vi "KeyboardSimulationForStringInput.vi"(0 "VI Reference In":refnum<vi>, 5 "Control Path":string, 7 "String Value":string, 11 "Error In":errorcluster) -> (4 "VI Reference Out":refnum<vi>, 15 "Error Out":errorcluster)   [LabVIEW 2016, in "Drona.lvlib" / "KeyboardSimulation.lvlib"]
doc: "Convert the input string value into key array and handle the actions configured for each of the keys in the control.\n\nThe input control name is given as a string , incase of path, use delimiters inbetween the path."
uses:
  KeyboardSimulation.lvlib
  typedef/VirtualKey.ctl
  typedef/Action.ctl
  user32.dll
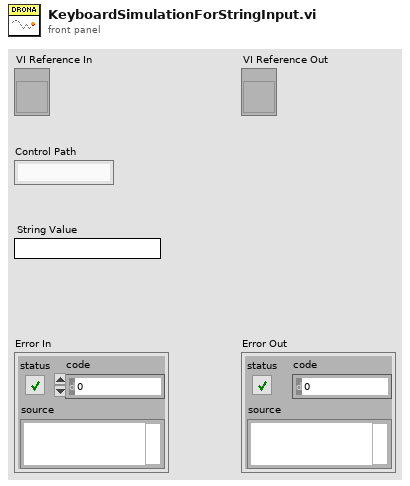
[diagram p1: front panel]
types:
  T1 = typedef "Drona.lvlib/KeyboardSimulation.lvlib/VirtualKey.ctl" = u8
  T2 = typedef "Drona.lvlib/KeyboardSimulation.lvlib/Action.ctl" = enum16{"Press", "Up", "Down"}
  T3 = cluster{"Key":T1, "Action":T2, "Delay (ms)":u32}[]
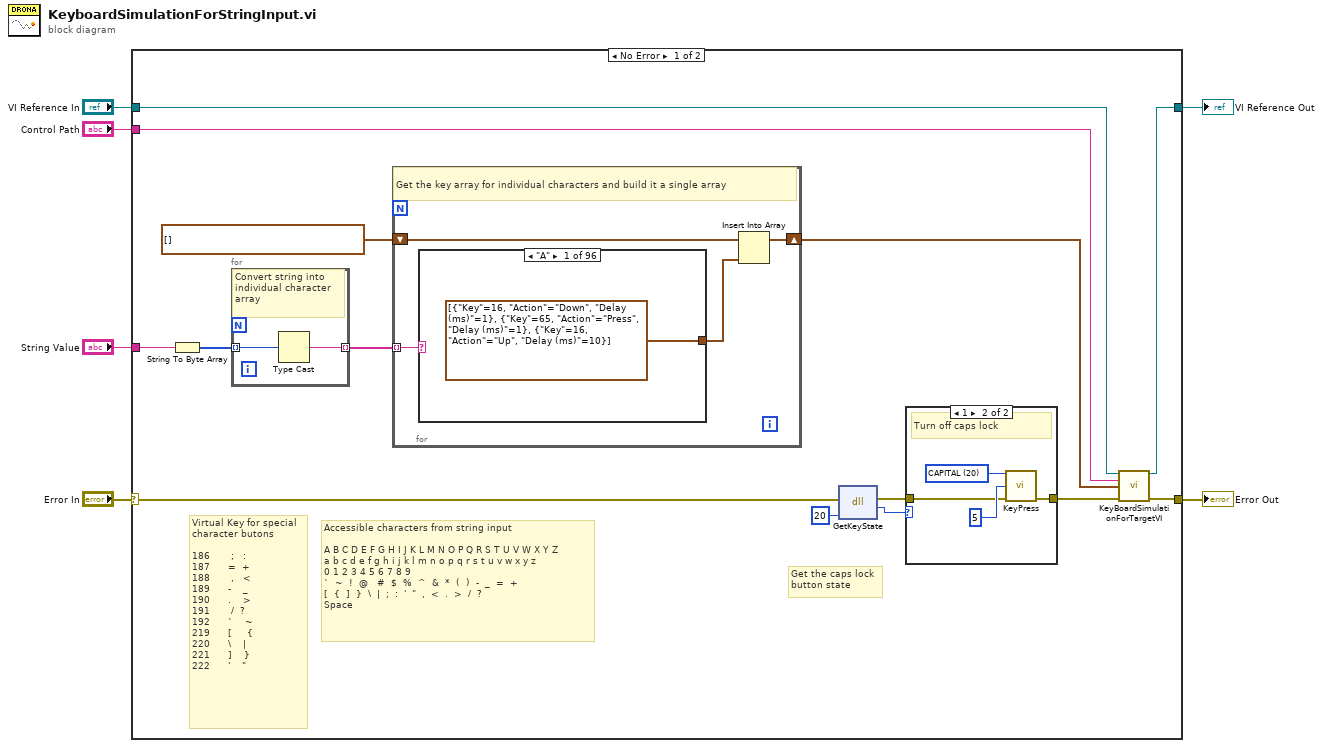
[diagram p0: block diagram]
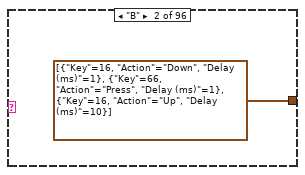
[diagram p2: hidden frame]
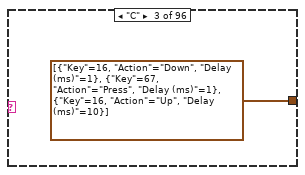
[diagram p3: hidden frame]
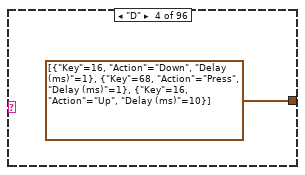
[diagram p4: hidden frame]
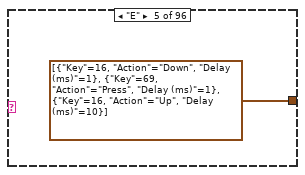
[diagram p5: hidden frame]
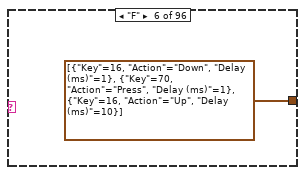
[diagram p6: hidden frame]
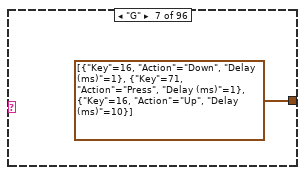
[diagram p7: hidden frame]
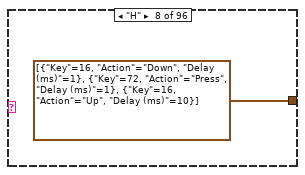
[diagram p8: hidden frame]
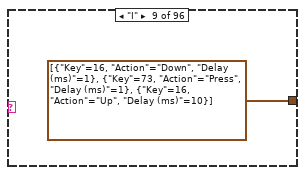
[diagram p9: hidden frame]
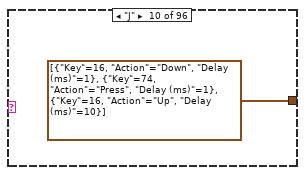
[diagram p10: hidden frame]
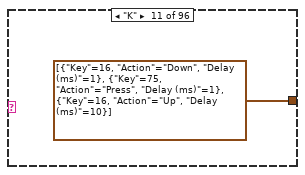
[diagram p11: hidden frame]
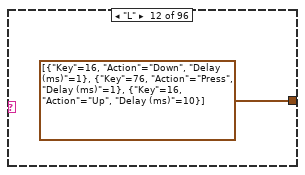
[diagram p12: hidden frame]
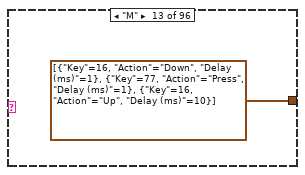
[diagram p13: hidden frame]
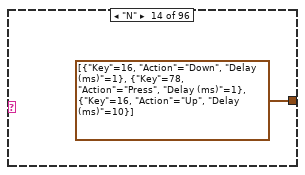
[diagram p14: hidden frame]
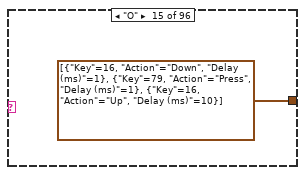
[diagram p15: hidden frame]
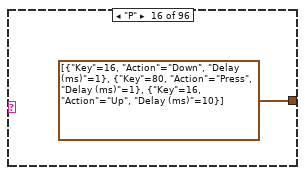
[diagram p16: hidden frame]
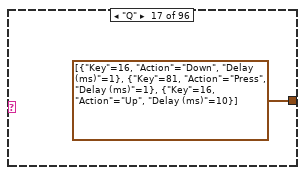
[diagram p17: hidden frame]
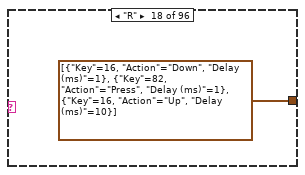
[diagram p18: hidden frame]
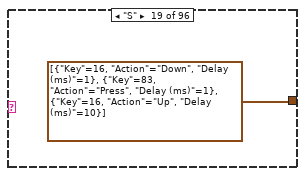
[diagram p19: hidden frame]
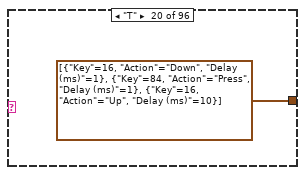
[diagram p20: hidden frame]
diagram:
  n1 = case shown="No Error" "Error In" {
    selector: "Error In" -> [w8 w128]
    tunnel: "String Value" -> [w17 _]
    tunnel: "VI Reference In" -> [w16 w129]
    tunnel: "Control Path" -> [w15 _]
    tunnel: [w14 w129] -> w2
    tunnel: [w13 w128] -> w1
    frame No Error {
      # "Virtual Key for special character butons\n\n186       ;   :\n187      =  +\n188       ,   <\n189      -    _\n190      .    >\n191       /  ?\n192      `    ~\n219      [     {\n220      \\    |\n221      ]    }\n222      '    \""
      # "Accessible characters from string input\n\nA B C D E F G H I J K L M N O P Q R S T U V W X Y Z \na b c d e f g h i j k l m n o p q r s t u v w x y z\n0 1 2 3 4 5 6 7 8 9\n`  ~  !  @   #  $  %  ^  &  *  (  )  -  _  =  + \n[  {  ]  }  \\  |  ;  :  '  \"  ,  <  .  >  /  ?\nSpace"
      # "Get the caps lock\nbutton state"
      n2 = String To Byte Array(string=w17) -> (unsigned byte array=w20:u8[])
      n3 = for {
        tunnel: w20 -> [w122] mode=indexing
        tunnel: [w121] -> w19 mode=indexing
        # "Convert string into individual character array"
        n4 = Type Cast(x=w122) -> (*(type *) &x=w121:string)  [unwired: 1 in]
      }
      n5 = for {
        tunnel: w19 -> [w22] mode=indexing
        shift-right: [w23] -> w7
        shift-left: T3 [] ("Key Array") -> [w24]
        # "Get the key array for individual characters and build it a single array"
        n6 = case shown="\"A\"" w22 {
          tunnel: [T3 [{"Key"=16, "Action"=enum."Down", "Delay (ms)"=1}, {"Key"=65, "Action"=enum."Press", "Delay (ms)"=1}, {"Key"=16, "Action"=enum."Up", "Delay (ms)"=10}] ("Key Array") T3 [{"Key"=16, "Action"=enum."Down", "Delay (ms)"=1}, {"Key"=66, "Action"=enum."Press", "Delay (ms)"=1}, {"Key"=16, "Action"=enum."Up", "Delay (ms)"=10}] ("Key Array") T3 [{"Key"=16, "Action"=enum."Down", "Delay (ms)"=1}, {"Key"=67, "Action"=enum."Press", "Delay (ms)"=1}, {"Key"=16, "Action"=enum."Up", "Delay (ms)"=10}] ("Key Array") T3 [{"Key"=16, "Action"=enum."Down", "Delay (ms)"=1}, {"Key"=68, "Action"=enum."Press", "Delay (ms)"=1}, {"Key"=16, "Action"=enum."Up", "Delay (ms)"=10}] ("Key Array") T3 [{"Key"=16, "Action"=enum."Down", "Delay (ms)"=1}, {"Key"=69, "Action"=enum."Press", "Delay (ms)"=1}, {"Key"=16, "Action"=enum."Up", "Delay (ms)"=10}] ("Key Array") T3 [{"Key"=16, "Action"=enum."Down", "Delay (ms)"=1}, {"Key"=70, "Action"=enum."Press", "Delay (ms)"=1}, {"Key"=16, "Action"=enum."Up", "Delay (ms)"=10}] ("Key Array") T3 [{"Key"=16, "Action"=enum."Down", "Delay (ms)"=1}, {"Key"=71, "Action"=enum."Press", "Delay (ms)"=1}, {"Key"=16, "Action"=enum."Up", "Delay (ms)"=10}] ("Key Array") T3 [{"Key"=16, "Action"=enum."Down", "Delay (ms)"=1}, {"Key"=72, "Action"=enum."Press", "Delay (ms)"=1}, {"Key"=16, "Action"=enum."Up", "Delay (ms)"=10}] ("Key Array") T3 [{"Key"=16, "Action"=enum."Down", "Delay (ms)"=1}, {"Key"=73, "Action"=enum."Press", "Delay (ms)"=1}, {"Key"=16, "Action"=enum."Up", "Delay (ms)"=10}] ("Key Array") T3 [{"Key"=16, "Action"=enum."Down", "Delay (ms)"=1}, {"Key"=74, "Action"=enum."Press", "Delay (ms)"=1}, {"Key"=16, "Action"=enum."Up", "Delay (ms)"=10}] ("Key Array") T3 [{"Key"=16, "Action"=enum."Down", "Delay (ms)"=1}, {"Key"=75, "Action"=enum."Press", "Delay (ms)"=1}, {"Key"=16, "Action"=enum."Up", "Delay (ms)"=10}] ("Key Array") T3 [{"Key"=16, "Action"=enum."Down", "Delay (ms)"=1}, {"Key"=76, "Action"=enum."Press", "Delay (ms)"=1}, {"Key"=16, "Action"=enum."Up", "Delay (ms)"=10}] ("Key Array") T3 [{"Key"=16, "Action"=enum."Down", "Delay (ms)"=1}, {"Key"=77, "Action"=enum."Press", "Delay (ms)"=1}, {"Key"=16, "Action"=enum."Up", "Delay (ms)"=10}] ("Key Array") T3 [{"Key"=16, "Action"=enum."Down", "Delay (ms)"=1}, {"Key"=78, "Action"=enum."Press", "Delay (ms)"=1}, {"Key"=16, "Action"=enum."Up", "Delay (ms)"=10}] ("Key Array") T3 [{"Key"=16, "Action"=enum."Down", "Delay (ms)"=1}, {"Key"=79, "Action"=enum."Press", "Delay (ms)"=1}, {"Key"=16, "Action"=enum."Up", "Delay (ms)"=10}] ("Key Array") T3 [{"Key"=16, "Action"=enum."Down", "Delay (ms)"=1}, {"Key"=80, "Action"=enum."Press", "Delay (ms)"=1}, {"Key"=16, "Action"=enum."Up", "Delay (ms)"=10}] ("Key Array") T3 [{"Key"=16, "Action"=enum."Down", "Delay (ms)"=1}, {"Key"=81, "Action"=enum."Press", "Delay (ms)"=1}, {"Key"=16, "Action"=enum."Up", "Delay (ms)"=10}] ("Key Array") T3 [{"Key"=16, "Action"=enum."Down", "Delay (ms)"=1}, {"Key"=82, "Action"=enum."Press", "Delay (ms)"=1}, {"Key"=16, "Action"=enum."Up", "Delay (ms)"=10}] ("Key Array") T3 [{"Key"=16, "Action"=enum."Down", "Delay (ms)"=1}, {"Key"=83, "Action"=enum."Press", "Delay (ms)"=1}, {"Key"=16, "Action"=enum."Up", "Delay (ms)"=10}] ("Key Array") T3 [{"Key"=16, "Action"=enum."Down", "Delay (ms)"=1}, {"Key"=84, "Action"=enum."Press", "Delay (ms)"=1}, {"Key"=16, "Action"=enum."Up", "Delay (ms)"=10}] ("Key Array") T3 [{"Key"=16, "Action"=enum."Down", "Delay (ms)"=1}, {"Key"=85, "Action"=enum."Press", "Delay (ms)"=1}, {"Key"=16, "Action"=enum."Up", "Delay (ms)"=10}] ("Key Array") T3 [{"Key"=16, "Action"=enum."Down", "Delay (ms)"=1}, {"Key"=86, "Action"=enum."Press", "Delay (ms)"=1}, {"Key"=16, "Action"=enum."Up", "Delay (ms)"=10}] ("Key Array") T3 [{"Key"=16, "Action"=enum."Down", "Delay (ms)"=1}, {"Key"=87, "Action"=enum."Press", "Delay (ms)"=1}, {"Key"=16, "Action"=enum."Up", "Delay (ms)"=10}] ("Key Array") T3 [{"Key"=16, "Action"=enum."Down", "Delay (ms)"=1}, {"Key"=88, "Action"=enum."Press", "Delay (ms)"=1}, {"Key"=16, "Action"=enum."Up", "Delay (ms)"=10}] ("Key Array") T3 [{"Key"=16, "Action"=enum."Down", "Delay (ms)"=1}, {"Key"=89, "Action"=enum."Press", "Delay (ms)"=1}, {"Key"=16, "Action"=enum."Up", "Delay (ms)"=10}] ("Key Array") T3 [{"Key"=16, "Action"=enum."Down", "Delay (ms)"=1}, {"Key"=90, "Action"=enum."Press", "Delay (ms)"=1}, {"Key"=16, "Action"=enum."Up", "Delay (ms)"=10}] ("Key Array") T3 [{"Key"=65, "Action"=enum."Press", "Delay (ms)"=10}] ("Key Array") T3 [{"Key"=66, "Action"=enum."Press", "Delay (ms)"=10}] ("Key Array") T3 [{"Key"=67, "Action"=enum."Press", "Delay (ms)"=10}] ("Key Array") T3 [{"Key"=68, "Action"=enum."Press", "Delay (ms)"=10}] ("Key Array") T3 [{"Key"=69, "Action"=enum."Press", "Delay (ms)"=10}] ("Key Array") T3 [{"Key"=70, "Action"=enum."Press", "Delay (ms)"=10}] ("Key Array") T3 [{"Key"=71, "Action"=enum."Press", "Delay (ms)"=10}] ("Key Array") T3 [{"Key"=72, "Action"=enum."Press", "Delay (ms)"=10}] ("Key Array") T3 [{"Key"=73, "Action"=enum."Press", "Delay (ms)"=10}] ("Key Array") T3 [{"Key"=74, "Action"=enum."Press", "Delay (ms)"=10}] ("Key Array") T3 [{"Key"=75, "Action"=enum."Press", "Delay (ms)"=10}] ("Key Array") T3 [{"Key"=76, "Action"=enum."Press", "Delay (ms)"=10}] ("Key Array") T3 [{"Key"=77, "Action"=enum."Press", "Delay (ms)"=10}] ("Key Array") T3 [{"Key"=78, "Action"=enum."Press", "Delay (ms)"=10}] ("Key Array") T3 [{"Key"=79, "Action"=enum."Press", "Delay (ms)"=10}] ("Key Array") T3 [{"Key"=80, "Action"=enum."Press", "Delay (ms)"=10}] ("Key Array") T3 [{"Key"=81, "Action"=enum."Press", "Delay (ms)"=10}] ("Key Array") T3 [{"Key"=82, "Action"=enum."Press", "Delay (ms)"=10}] ("Key Array") T3 [{"Key"=83, "Action"=enum."Press", "Delay (ms)"=10}] ("Key Array") T3 [{"Key"=84, "Action"=enum."Press", "Delay (ms)"=10}] ("Key Array") T3 [{"Key"=85, "Action"=enum."Press", "Delay (ms)"=10}] ("Key Array") T3 [{"Key"=86, "Action"=enum."Press", "Delay (ms)"=10}] ("Key Array") T3 [{"Key"=87, "Action"=enum."Press", "Delay (ms)"=10}] ("Key Array") T3 [{"Key"=88, "Action"=enum."Press", "Delay (ms)"=10}] ("Key Array") T3 [{"Key"=89, "Action"=enum."Press", "Delay (ms)"=10}] ("Key Array") T3 [{"Key"=90, "Action"=enum."Press", "Delay (ms)"=10}] ("Key Array") T3 [{"Key"=48, "Action"=enum."Press", "Delay (ms)"=10}] ("Key Array") T3 [{"Key"=49, "Action"=enum."Press", "Delay (ms)"=10}] ("Key Array") T3 [{"Key"=50, "Action"=enum."Press", "Delay (ms)"=10}] ("Key Array") T3 [{"Key"=51, "Action"=enum."Press", "Delay (ms)"=10}] ("Key Array") T3 [{"Key"=52, "Action"=enum."Press", "Delay (ms)"=10}] ("Key Array") T3 [{"Key"=53, "Action"=enum."Press", "Delay (ms)"=10}] ("Key Array") T3 [{"Key"=54, "Action"=enum."Press", "Delay (ms)"=10}] ("Key Array") T3 [{"Key"=55, "Action"=enum."Press", "Delay (ms)"=10}] ("Key Array") T3 [{"Key"=56, "Action"=enum."Press", "Delay (ms)"=10}] ("Key Array") T3 [{"Key"=57, "Action"=enum."Press", "Delay (ms)"=10}] ("Key Array") T3 [{"Key"=16, "Action"=enum."Down", "Delay (ms)"=1}, {"Key"=49, "Action"=enum."Press", "Delay (ms)"=1}, {"Key"=16, "Action"=enum."Up", "Delay (ms)"=10}] ("Key Array") T3 [{"Key"=16, "Action"=enum."Down", "Delay (ms)"=1}, {"Key"=50, "Action"=enum."Press", "Delay (ms)"=1}, {"Key"=16, "Action"=enum."Up", "Delay (ms)"=10}] ("Key Array") T3 [{"Key"=16, "Action"=enum."Down", "Delay (ms)"=1}, {"Key"=51, "Action"=enum."Press", "Delay (ms)"=1}, {"Key"=16, "Action"=enum."Up", "Delay (ms)"=10}] ("Key Array") T3 [{"Key"=16, "Action"=enum."Down", "Delay (ms)"=1}, {"Key"=52, "Action"=enum."Press", "Delay (ms)"=1}, {"Key"=16, "Action"=enum."Up", "Delay (ms)"=10}] ("Key Array") T3 [{"Key"=16, "Action"=enum."Down", "Delay (ms)"=1}, {"Key"=53, "Action"=enum."Press", "Delay (ms)"=1}, {"Key"=16, "Action"=enum."Up", "Delay (ms)"=10}] ("Key Array") T3 [{"Key"=16, "Action"=enum."Down", "Delay (ms)"=1}, {"Key"=54, "Action"=enum."Press", "Delay (ms)"=1}, {"Key"=16, "Action"=enum."Up", "Delay (ms)"=10}] ("Key Array") T3 [{"Key"=16, "Action"=enum."Down", "Delay (ms)"=1}, {"Key"=55, "Action"=enum."Press", "Delay (ms)"=1}, {"Key"=16, "Action"=enum."Up", "Delay (ms)"=10}] ("Key Array") T3 [{"Key"=16, "Action"=enum."Down", "Delay (ms)"=1}, {"Key"=56, "Action"=enum."Press", "Delay (ms)"=1}, {"Key"=16, "Action"=enum."Up", "Delay (ms)"=10}] ("Key Array") T3 [{"Key"=16, "Action"=enum."Down", "Delay (ms)"=1}, {"Key"=57, "Action"=enum."Press", "Delay (ms)"=1}, {"Key"=16, "Action"=enum."Up", "Delay (ms)"=10}] ("Key Array") T3 [{"Key"=16, "Action"=enum."Down", "Delay (ms)"=1}, {"Key"=48, "Action"=enum."Press", "Delay (ms)"=1}, {"Key"=16, "Action"=enum."Up", "Delay (ms)"=10}] ("Key Array") T3 [{"Key"=186, "Action"=enum."Press", "Delay (ms)"=10}] ("Key Array") T3 [{"Key"=16, "Action"=enum."Down", "Delay (ms)"=1}, {"Key"=186, "Action"=enum."Press", "Delay (ms)"=1}, {"Key"=16, "Action"=enum."Up", "Delay (ms)"=10}] ("Key Array") T3 [{"Key"=187, "Action"=enum."Press", "Delay (ms)"=10}] ("Key Array") T3 [{"Key"=16, "Action"=enum."Down", "Delay (ms)"=1}, {"Key"=187, "Action"=enum."Press", "Delay (ms)"=1}, {"Key"=16, "Action"=enum."Up", "Delay (ms)"=10}] ("Key Array") T3 [{"Key"=188, "Action"=enum."Press", "Delay (ms)"=10}] ("Key Array") T3 [{"Key"=16, "Action"=enum."Down", "Delay (ms)"=1}, {"Key"=188, "Action"=enum."Press", "Delay (ms)"=1}, {"Key"=16, "Action"=enum."Up", "Delay (ms)"=10}] ("Key Array") T3 [{"Key"=189, "Action"=enum."Press", "Delay (ms)"=10}] ("Key Array") T3 [{"Key"=16, "Action"=enum."Down", "Delay (ms)"=1}, {"Key"=189, "Action"=enum."Press", "Delay (ms)"=1}, {"Key"=16, "Action"=enum."Up", "Delay (ms)"=10}] ("Key Array") T3 [{"Key"=190, "Action"=enum."Press", "Delay (ms)"=10}] ("Key Array") T3 [{"Key"=16, "Action"=enum."Down", "Delay (ms)"=1}, {"Key"=190, "Action"=enum."Press", "Delay (ms)"=1}, {"Key"=16, "Action"=enum."Up", "Delay (ms)"=10}] ("Key Array") T3 [{"Key"=191, "Action"=enum."Press", "Delay (ms)"=10}] ("Key Array") T3 [{"Key"=16, "Action"=enum."Down", "Delay (ms)"=1}, {"Key"=191, "Action"=enum."Press", "Delay (ms)"=1}, {"Key"=16, "Action"=enum."Up", "Delay (ms)"=10}] ("Key Array") T3 [{"Key"=192, "Action"=enum."Press", "Delay (ms)"=10}] ("Key Array") T3 [{"Key"=16, "Action"=enum."Down", "Delay (ms)"=1}, {"Key"=192, "Action"=enum."Press", "Delay (ms)"=1}, {"Key"=16, "Action"=enum."Up", "Delay (ms)"=10}] ("Key Array") T3 [{"Key"=219, "Action"=enum."Press", "Delay (ms)"=10}] ("Key Array") T3 [{"Key"=16, "Action"=enum."Down", "Delay (ms)"=1}, {"Key"=219, "Action"=enum."Press", "Delay (ms)"=1}, {"Key"=16, "Action"=enum."Up", "Delay (ms)"=10}] ("Key Array") T3 [{"Key"=220, "Action"=enum."Press", "Delay (ms)"=10}] ("Key Array") T3 [{"Key"=16, "Action"=enum."Down", "Delay (ms)"=1}, {"Key"=220, "Action"=enum."Press", "Delay (ms)"=1}, {"Key"=16, "Action"=enum."Up", "Delay (ms)"=10}] ("Key Array") T3 [{"Key"=221, "Action"=enum."Press", "Delay (ms)"=10}] ("Key Array") T3 [{"Key"=16, "Action"=enum."Down", "Delay (ms)"=1}, {"Key"=221, "Action"=enum."Press", "Delay (ms)"=1}, {"Key"=16, "Action"=enum."Up", "Delay (ms)"=10}] ("Key Array") T3 [{"Key"=222, "Action"=enum."Press", "Delay (ms)"=10}] ("Key Array") T3 [{"Key"=16, "Action"=enum."Down", "Delay (ms)"=1}, {"Key"=222, "Action"=enum."Press", "Delay (ms)"=1}, {"Key"=16, "Action"=enum."Up", "Delay (ms)"=10}] ("Key Array") T3 [{"Key"=32, "Action"=enum."Press", "Delay (ms)"=10}] ("Key Array") T3 [] ("Key Array")] -> w21
          frame "A" {
          }
          frame "B" {
          }
          frame "C" {
          }
          frame "D" {
          }
          frame "E" {
          }
          frame "F" {
          }
          frame "G" {
          }
          frame "H" {
          }
          frame "I" {
          }
          frame "J" {
          }
          frame "K" {
          }
          frame "L" {
          }
          frame "M" {
          }
          frame "N" {
          }
          frame "O" {
          }
          frame "P" {
          }
          frame "Q" {
          }
          frame "R" {
          }
          frame "S" {
          }
          frame "T" {
          }
          frame "U" {
          }
          frame "V" {
          }
          frame "W" {
          }
          frame "X" {
          }
          frame "Y" {
          }
          frame "Z" {
          }
          frame "a" {
          }
          frame "b" {
          }
          frame "c" {
          }
          frame "d" {
          }
          frame "e" {
          }
          frame "f" {
          }
          frame "g" {
          }
          frame "h" {
          }
          frame "i" {
          }
          frame "j" {
          }
          frame "k" {
          }
          frame "l" {
          }
          frame "m" {
          }
          frame "n" {
          }
          frame "o" {
          }
          frame "p" {
          }
          frame "q" {
          }
          frame "r" {
          }
          frame "s" {
          }
          frame "t" {
          }
          frame "u" {
          }
          frame "v" {
          }
          frame "w" {
          }
          frame "x" {
          }
          frame "y" {
          }
          frame "z" {
          }
          frame "0" {
          }
          frame "1" {
          }
          frame "2" {
          }
          frame "3" {
          }
          frame "4" {
          }
          frame "5" {
          }
          frame "6" {
          }
          frame "7" {
          }
          frame "8" {
          }
          frame "9" {
          }
          frame "!" {
          }
          frame "@" {
          }
          frame "#" {
          }
          frame "$" {
          }
          frame "%" {
          }
          frame "^" {
          }
          frame "&" {
          }
          frame "*" {
          }
          frame "(" {
          }
          frame ")" {
          }
          frame ";" {
          }
          frame ":" {
          }
          frame "=" {
          }
          frame "+" {
          }
          frame "," {
          }
          frame "<" {
          }
          frame "-" {
          }
          frame "_" {
          }
          frame "." {
          }
          frame ">" {
          }
          frame "/" {
          }
          frame "?" {
          }
          frame "`" {
          }
          frame "~" {
          }
          frame "[" {
          }
          frame "{" {
          }
          frame "\\" {
          }
          frame "|" {
          }
          frame "]" {
          }
          frame "}" {
          }
          frame "'" {
          }
          frame "\"" {
          }
          frame " " {
          }
          frame Default {
          }
        }
        n7 = Insert Into Array(array=w24, new element=w21) -> (w23:T3)  [unwired: 1 in]
      }
      n8 = dll-call lib="user32.dll" fn="GetKeyState"(error in=w8, "arg"=u8 20 ("Virtual Key")) -> (error out=w9:errorcluster, "return type"=w10:u8)  [unwired: 3 in, 1 out]
      n9 = case shown="1" w10 {
        tunnel: [w123 w127] -> w12
        tunnel: w9 -> [w123 w124]
        frame 0, Default {
          # "Caps lock is off"
        }
        frame 1 {
          w125 = T1 20 items=["LBUTTON"=1, "RBUTTON"=2, "CANCEL"=3, "MBUTTON"=4, "BACKSPACE"=8, "TAB"=9, "CLEAR"=12, "ENTER"=13, "SHIFT"=16, "CTRL"=17, "ALT"=18, "PAUSE"=19, "CAPITAL"=20, "ESCAPE"=27, "SPACE"=32, "PAGEUP"=33, "PAGEDOWN"=34, "END"=35, "HOME"=36, "LEFTARROW"=37, "UPARROW"=38, "RIGHTARROW"=39, "DOWNARROW"=40, "SELECT"=41, "PRINT"=42, "EXECUTE"=43, "PRINTSCREEN"=44, "INSERT"=45, "DELETE"=46, "HELP"=47, "0"=48, "1"=49, "2"=50, "3"=51, "4"=52, "5"=53, "6"=54, "7"=55, "8"=56, "9"=57, "A"=65, "B"=66, "C"=67, "D"=68, "E"=69, "F"=70, "G"=71, "H"=72, "I"=73, "J"=74, "K"=75, "L"=76, "M"=77, "N"=78, "O"=79, "P"=80, "Q"=81, "R"=82, "S"=83, "T"=84, "U"=85, "V"=86, "W"=87, "X"=88, "Y"=89, "Z"=90, "LWIN"=91, "RWIN"=92, "APPS"=93, "NUMPAD0"=96, "NUMPAD1"=97, "NUMPAD2"=98, "NUMPAD3"=99, "NUMPAD4"=100, "NUMPAD5"=101, "NUMPAD6"=102, "NUMPAD7"=103, "NUMPAD8"=104, "NUMPAD9"=105, "MULTIPLY"=106, "ADD"=107, "SEPERATOR"=108, "SUBTRACT"=109, "DECIMAL"=110, "DIVIDE"=111, "F1"=112, "F2"=113, "F3"=114, "F4"=115, "F5"=116, "F6"=117, "F7"=118, "F8"=119, "F9"=120, "F10"=121, "F11"=122, "F12"=123, "F13"=124, "F14"=125, "F15"=126, "F16"=127, "F17"=128, "F18"=129, "F19"=130, "F20"=131, "F21"=132, "F22"=133, "F23"=134, "F24"=135, "NUMLOCK"=144, "SCROLL"=145, "LSHIFT"=160, "RSHIFT"=161, "LCTRL"=162, "RCTRL"=163, "LALT"=164, "RALT"=165, "VOLMUTE"=173, "VOLDOWN"=174, "VOLUP"=175, ";    :"=186, "=   +"=187, ",    <"=188, "-    _"=189, ".    >"=190, "/    ?"=191, "`    ~"=192, "[    {"=219, "\\    |"=220, "]    }"=221, "'    \""=222] ("Virtual Key")
          # "Turn off caps lock"
          n10 = call "KeyPress.vi"("Virtual Key"=w125, "Millis"=u32 5, "error in"=w124) -> ("error out"=w127:errorcluster)  [unwired: 12 in]
        }
      }
      n11 = call "KeyBoardSimulationForTargetVI.vi"("VI Reference In"=w16, "Control Path"=w15, "Key Array"=w7, "error In"=w12) -> ("VI Reference Out"=w14:refnum<vi>, "error IO"=w13:errorcluster)  [unwired: 10 in]
    }
    frame Error {
    }
  }
  "VI Reference Out" <- w2
  "Error Out" <- w1
